vi "RT Main.vi"() -> ()   [LabVIEW 2021]
doc: "This example shows how to debounce a digital signal acquired from a push button switch."
uses:
  <vilib>/Waveform/DWDTOps.llb/DWDT Boolean Array to Digital.vi
  <vilib>/myRIO/Instrument Drivers/Utilities/Utilities.lvlib
  <vilib>/Platform/TimedLoop/XDataNode/XDataNode.xnode
  <vilib>/Platform/TimedLoop/XDataNode/nitl_modes.ctl
  <vilib>/Platform/TimedLoop/XDataNode/XDNodeRunTimeDep.lvlib
  <vilib>/Platform/TimedLoop/XDataNode/wakeup.ctl
  <vilib>/Platform/TimedLoop/XDataNode/timing_clust.ctl
  <vilib>/myRIO/Express VI/Onboard IO/DI/DI Express VI.xnode
  <vilib>/myRIO/Instrument Drivers/Onboard IO/DIO/vis/Read.vi
  <vilib>/myRIO/Instrument Drivers/Onboard IO/DIO/DIO.lvlib
  <vilib>/myRIO/Common/Instrument Driver Framework/myRIO v1.0/DIO/typedefs/DIO Channels Enum.ctl
  <vilib>/myRIO/Common/Instrument Driver Framework/myRIO v1.0/DIO/typedefs/DIO Channels List.ctl
  <vilib>/myRIO/Common/Instrument Driver Framework/Utilities/typedefs/Generic FPGA Reference.ctl
  <vilib>/myRIO/Common/Instrument Driver Framework/Utilities/typedefs/myRIO v1.0 Reference.ctl
  <vilib>/myRIO/Common/Instrument Driver Framework/Utilities/typedefs/Hardware Version Enum.ctl
  <vilib>/myRIO/Common/Instrument Driver Framework/Utilities/typedefs/myRIO Generic Hardware Reference.ctl
  <vilib>/myRIO/Instrument Drivers/Onboard IO/DIO/typedefs/DIO Reference.ctl
  <vilib>/myRIO/Instrument Drivers/Onboard IO/DIO/vis/myRIO DIO Open.xnode
  <vilib>/myRIO/Common/Instrument Driver Framework/Utilities/vis/Is FPGA Ref Available.vi
  <vilib>/myRIO/Common/Instrument Driver Framework/myRIO v1.0/DIO/vis/myRIO v1.1 Open DIO.vi
  <vilib>/userdefined/High Color/nirio_resource_hc.ctl
panel:
  out "error out":errorcluster
  out "Debounced Signal":digitalwaveform(graph)
  out "Original Signal":digitalwaveform(graph)
  in  "Stop":bool
  # "Overview: This example shows how to debounce a digital signal acquired from a push button switch.\nInstructions:\n1. Connect an external push button switch to DIO0 on connector A.\n2. Check the myRIO target IP Address in the project and make sure the target IP Address is correct.\n3. Run this VI.\n4. Depending on the quality of the push button switch, you may or may not see jitter."
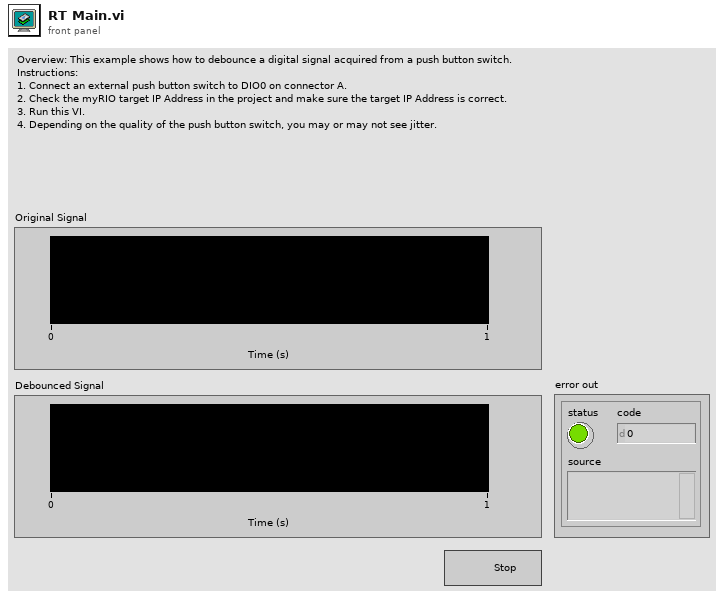
[diagram p1: front panel]
types:
  T1 = typedef "DIO.lvlib/DIO Reference.ctl" = cluster{"myRIO Reference":T2, "DIO Channels List":T6}
  T2 = typedef "myRIO Generic Hardware Reference.ctl" = cluster{"myRIO Model":T3, "myRIO Hardware Reference":T4}
  T3 = typedef "Hardware Version Enum.ctl" = enum16{"Unknown", "myRIO-1900", "myRIO-1950", "roboRIO", "NI ELVIS RIO CM", "ELVIS III"}
  T4 = typedef "myRIO v1.0 Reference.ctl" = cluster{"Generic FPGA Reference":T5, "Allow multiple opens":bool}
  T5 = typedef "Generic FPGA Reference.ctl" = refnum<k20>
  T6 = typedef "DIO Channels List.ctl" = T7[]
  T7 = typedef "DIO Channels Enum.ctl" = enum16{"Not Connected", "C/DIO0", "C/DIO1", "C/DIO2", "C/DIO3", "C/DIO4", "C/DIO5", "C/DIO6", "C/DIO7", "A/DIO0", "A/DIO1", "A/DIO2", "A/DIO3", "A/DIO4", "A/DIO5", "A/DIO6", "A/DIO7", "A/DIO8", "A/DIO9", "A/DIO10", "A/DIO11", "A/DIO12", "A/DIO13", "A/DIO14", "A/DIO15", "A/DIO16", "A/DIO17", "A/DIO18", "A/DIO19", "B/DIO0", "B/DIO1", "B/DIO2", "B/DIO3", "B/DIO4", "B/DIO5", "B/DIO6", "B/DIO7", "B/DIO8", "B/DIO9", "B/DIO10", "B/DIO11", "B/DIO12", "B/DIO13", "B/DIO14", "B/DIO15", "B/DIO16", "B/DIO17", "B/DIO18", "B/DIO19", "LED0", "LED1", "LED2", "LED3", "Button0", "DIO/DIO0", "DIO/DIO1", "DIO/DIO2", "DIO/DIO3", "DIO/DIO4", "DIO/DIO5", "DIO/DIO6", "DIO/DIO7", "DIO/DIO8", "DIO/DIO9", "SPI/CS0", "SPI/CS1", "SPI/CS2", "SPI/CS3", "LED RADIO (Green)", "LED RADIO (Red)", "LED COMM (Green)", "LED COMM (Red)", "LED MODE (Green)", "LED MODE (Red)"}
  T8 = typedef "nirio_resource_hc.ctl" = tag
  T9 = typedef "XDNodeRunTimeDep.lvlib/timing_clust.ctl" = cluster{"Expected End [f-1]":u64, "Actual End [f-1]":u64, "Finished Late? [f-1]":bool, "Expected End [i-1]":u64, "Actual End [i-1]":u64, "Finished Late? [i-1]":bool, "Expected Start [i]":u64, "Actual Start [i]":u64, "Expected Start [f]":u64, "Actual Start [f]":u64, "Source Name":string, "Structure Name":string, "Period":i64, "Deadline":i64, "Offset":i64, "Start":i64, "Priority":i32, "Timeout":i32, "Mode":T10, "Wakeup Reason":T11, "Error":errorcluster, "Source Type":string, "Secondary Source Type":string, "Global End Time":u64, "Global Start Time":u64, "Frame Duration":u64, "Iteration Duration":u64, "Assigned CPU":i32, "I/O Scan Engine Mode":u32}
  T10 = typedef "XDNodeRunTimeDep.lvlib/nitl_modes.ctl" = enum32{"No Change", "Process missed periods, maintain original phase", "Discard missed periods, maintain original phase", "Process missed periods, ignore original phase", "Discard missed periods, ignore original phase"}
  T11 = typedef "XDNodeRunTimeDep.lvlib/wakeup.ctl" = enum32{"Normal", "Aborted", "Asynchronous wakeup", "Timing source error", "Timed loop error", "Timeout"}
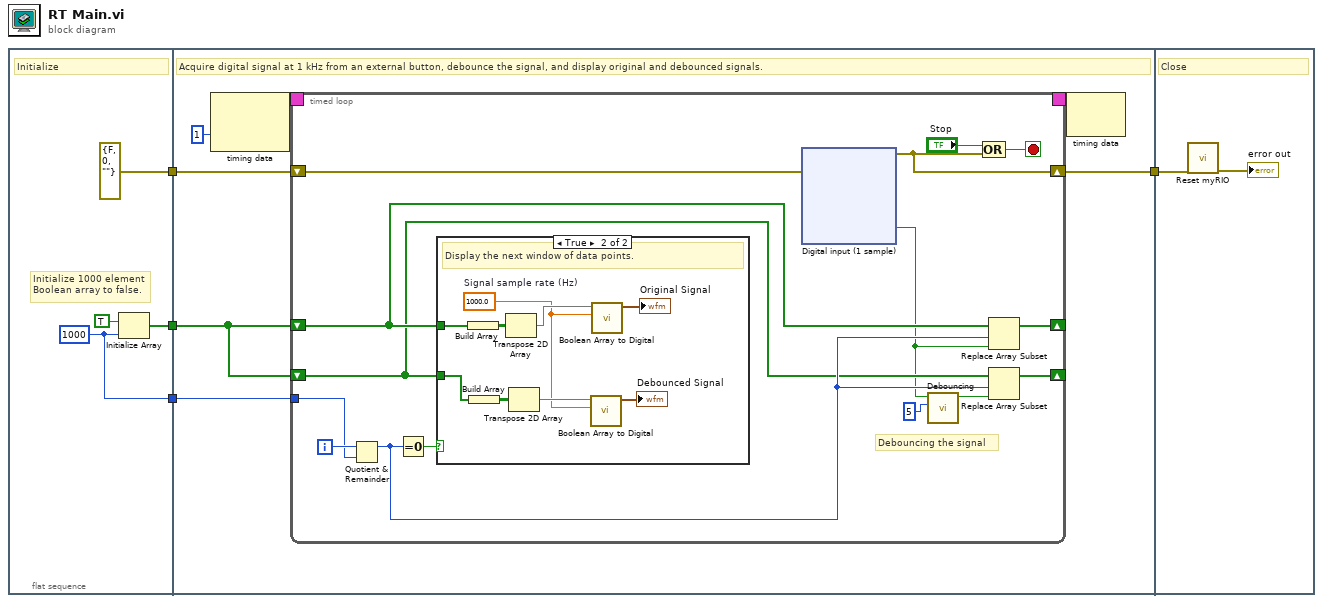
[diagram p0: block diagram]
diagram:
  n1 = flat-sequence {
    tunnel: [errorcluster {"status"=FALSE, "code"=0, "source"=""} ("error in (no error)")] -> w4
    tunnel: [w6] -> w3
    tunnel: [w5] -> w1
    tunnel: w4 -> [w12]
    tunnel: w3 -> [w13]
    tunnel: [w11] -> w2
    tunnel: w1 -> [w9]
    tunnel: w2 -> [w82]
    frame #0 {
      w5 = 1000 ("dimension size")
      # "Initialize 1000 element\nBoolean array to false."
      # "Initialize"
      n2 = Initialize Array(TRUE ("boolean ()"), w5) -> (w6:bool[])
    }
    frame #1 {
      # "Acquire digital signal at 1 kHz from an external button, debounce the signal, and display original and debounced signals."
      n3 = node-c288(i64 1 ("Period")) -> (w15:T9)  [unwired: 1 in]
      n4 = timed-loop {
        shift-right: [w17] -> w11
        shift-left: w12 -> [w18]
        shift-right: [w23] -> _
        shift-left: w13 -> [w20]
        shift-right: [w22] -> _
        shift-left: w13 -> [w19]
        timing: w15 -> [_]
        timing-out: [_] -> w14
        tunnel: w9 -> [w24]
        i -> [w25]
        stop <- w30 stop-if-true
        # "Debouncing the signal"
        n5 = Quotient & Remainder(x=w25, y=w24) -> (x-y*floor(x/y)=w21:i32)  [unwired: 1 out]
        n6 = Equal To 0?(x=w21) -> (x = 0?=w26:bool)
        n7 = case shown="True" w26 {
          tunnel: w19 -> [_ w68]
          tunnel: w20 -> [_ w67]
          frame False {
          }
          frame True {
            w66 = 1000.0  # Signal sample rate (Hz)
            # "Display the next window of data points."
            n8 = Build Array(w67) -> (w72:bool[][])
            n9 = Build Array(w68) -> (w70:bool[][])
            n10 = Transpose 2D Array(2D array=w72) -> (transposed array=w71:bool[][])
            n11 = Transpose 2D Array(2D array=w70) -> (transposed array=w69:bool[][])
            n12 = call-poly <vilib>:"Boolean Array to Digital.vi"("sample rate"=w66, "boolean array"=w69) -> ("digital waveform"=→"Debounced Signal":digitalwaveform)  [unwired: 8 in, 1 out]
            n13 = call-poly <vilib>:"Boolean Array to Digital.vi"("sample rate"=w66, "boolean array"=w71) -> ("digital waveform"=→"Original Signal":digitalwaveform)  [unwired: 8 in, 1 out]
          }
        }
        n14 = xnode "Digital input (1 sample)"("error in (no error)"=w18) -> ("A/DIO0 (Pin 11)"=w16:bool, "error out"=w17:errorcluster)
        n15 = call "Debouncing.vi"("Cycles to Filter"=u16 5, "New Input Signal"=w16) -> ("New Signal"=w27:bool)  [unwired: 8 in, 1 out]
        n16 = Compound Arithmetic op=OR("Stop", w17) -> (w30:bool)
        n17 = Replace Array Subset(array=w20, new element=w16, index=w21) -> (w23:bool[])
        n18 = Replace Array Subset(array=w19, new element=w27, index=w21) -> (w22:bool[])
      }
      n19 = node-c288(w14) -> ()  [unwired: 1 out]
    }
    frame #2 {
      # "Close"
      n20 = call <vilib>:"Reset myRIO.vi"("error in (no error)"=w82) -> ("error out"=→"error out":errorcluster)  [unwired: 10 in]
    }
  }
